vi "Configure Edge Trigger Source.vi"(0 "CS++Scope":refnum<class "CS++Scope.lvclass">, 5 "trigger source (CHANNEL1)":string(combo)="CHANNEL1" caption="trigger source (\"CHANNEL1\")", 7 "trigger slope (Positive)":i32(ring)=1 items=["Positive"=1, "Negative"=0], 9 "trigger level  (0.0 V)":dbl[unit] format="%.3f", 11 "error in (no error)":errorcluster) -> (4 "CS++Scope out":refnum<class "CS++Scope.lvclass">, 15 "error out":errorcluster)   [LabVIEW 2015, in "CS++Scope.lvlib" / "CS++Scope.lvclass"]
doc: "This VI configures the edge trigger. An edge trigger occurs when the trigger signal passes through the voltage threshold that you specify with the Trigger Level parameter and has the slope that you specify with the Trigger Slope parameter. \n\nNotes:\n (1) This VI affects instrument behavior only if the trigger type is\n IVISCOPE_VAL_EDGE_TRIGGER. Call the IviScope Configure Trigger and\n IviScope Configure Trigger Coupling VIs to set the trigger type and trigger coupling\n before calling this VI.\n (2) If the trigger source is one of the analog input channels, you must configure\n the vertical range, vertical offset, vertical coupling, probe attenuation, and the\n maximum input frequency before calling this VI."
uses:
  CS++Scope.lvclass
  CSPP_Core/Classes/CS++ProcessVariables/ProcessVariable/PV.lvclass
  PV-Enum.ctl
  CS++Scope.lvclass/CS++Scope.ctl
  CSPP_Core/Classes/CS++ProcessVariables/ProcessVariable/PV.lvclass/PV.ctl
  CSPP_Core/Classes/CS++ProcessVariables/ProcessVariable/Write Data.vi
  CSPP_Core/Classes/CS++ProcessVariables/ProcessVariable/Write Timestamp.vi
  CSPP_Core/Classes/CS++ProcessVariables/ProcessVariable/Write Quality.vi
  CSPP_Core/Classes/CS++ProcessVariables/ProcessVariable/Write status.vi
  CSPP_Core/Classes/CS++ProcessVariables/PVConnection/PVConnection.lvclass
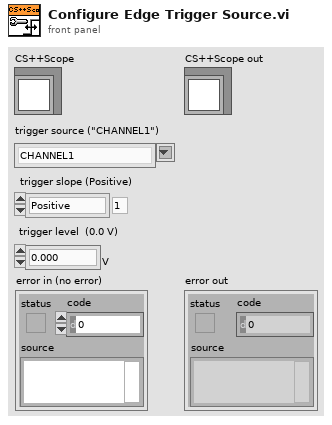
[diagram p1: front panel]
types:
  T1 = typedef "CS++Scope.lvlib/CS++Scope.lvclass/PV-Enum.ctl" = enum16{"ActualSampleRate", "TimePerRecord", "AcquisitionStartTime", "TriggerLevel", "GlitchWidth", "LowReference", "MidReference", "HighReference", "RuntLowThreshold", "RuntHighThreshold", "TriggerHoldoff", "WidthLowThreshold", "WidthHighThreshold", "AcquisitionStatus", "ActualRecordLength", "ActualSampleMode", "ACLineTriggerSlope", "MinRecordLength", "AcquisitionType", "TriggerSlope", "GlitchCondition", "GlitchPolarity", "InterpolationMethod", "NumberOfAverages", "NumberOfEnvelopes", "TriggerType", "TriggerCoupling", "TriggerModifier", "TVLineNumber", "TVEvent", "TVTriggerPolarity", "TVSignalFormat", "WidthCondition", "WidthPolarity", "MeasurementDone", "ContinousAcquisition", "TriggerSource", "Waveform", "ActualTimeIncrement"}
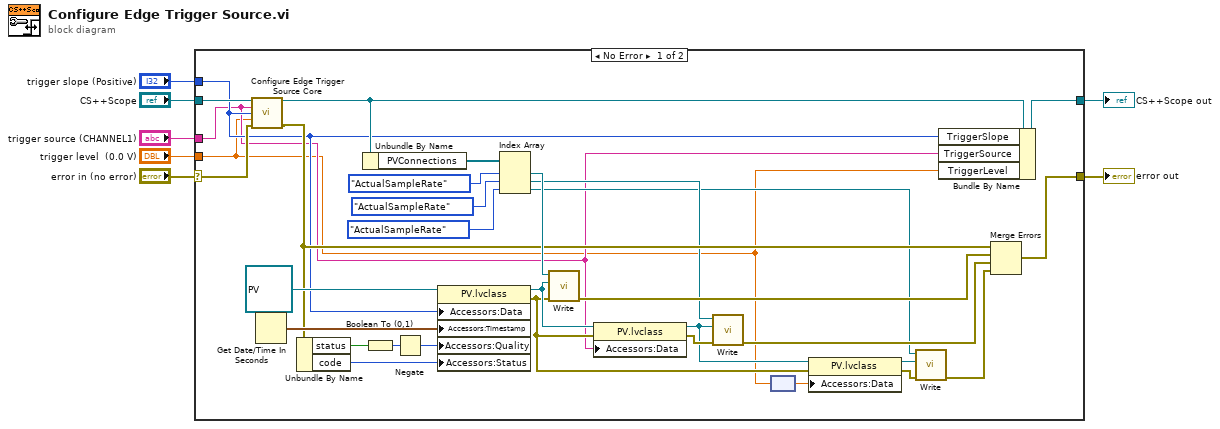
[diagram p0: block diagram]
diagram:
  n1 = case shown="No Error" "error in (no error)" {
    selector: "error in (no error)" -> [w13 w41]
    tunnel: [w12 w41] -> w6
    tunnel: [w14 w40] -> w2
    tunnel: "CS++Scope" -> [w15 w40]
    tunnel: "trigger source (CHANNEL1)" -> [w10 _]
    tunnel: "trigger level  (0.0 V)" -> [w9 _]
    tunnel: "trigger slope (Positive)" -> [w11 _]
    frame No Error {
      n2 = call-dynamic "Configure Edge Trigger Source Core.vi"("CS++Scope"=w15, "trigger source (CHANNEL1)"=w10, "trigger slope (Positive)"=w11, "trigger level  (0.0 V)"=w9, "error in (no error)"=w13) -> ("CS++Scope out"=w29:refnum<class "CS++Scope.lvclass">, "error out"=w28:errorcluster)  [unwired: 9 in]
      n3 = Get Date/Time In Seconds() -> (seconds since 1Jan1904=w34:timestamp)
      n4 = Unbundle By Name(w28) -> ("status"=w37:bool, "code"=w38:i32)
      n5 = Unbundle By Name(w29) -> ("PVConnections"=w33:refnum<class "PVConnection.lvclass">[])
      n6 = Boolean To (0,1)(Boolean=w37) -> (0, 1=w36:i16)
      n7 = Negate(x=w36) -> (-x=w35:i16)
      n8 = property class="PV.lvclass"(reference=refnum<class "PV.lvclass"> refnum ("CS++ProcessVariables.lvlib:PV.lvclass"), "Accessors:Data"=w11, "Accessors:Timestamp"=w34, "Accessors:Quality"=w35, "Accessors:Status"=w38) -> (reference out=w23:refnum<class "PV.lvclass">, error out=w19:errorcluster)  [unwired: 1 in]
      n9 = Index Array(array=w33, index #1=PV-Enum."ActualSampleRate" ("PV-Enum"), index #2=PV-Enum."ActualSampleRate" ("PV-Enum"), index #3=PV-Enum."ActualSampleRate" ("PV-Enum")) -> (element #1=w31:refnum<class "PVConnection.lvclass">, element #2=w21:refnum<class "PVConnection.lvclass">, element #3=w17:refnum<class "PVConnection.lvclass">)
      n10 = call "Write.vi"("error in (no error)"=w19, "PV"=w23, "PVConnection in"=w31) -> ("error out"=w30:errorcluster)  [unwired: 7 in, 1 out]
      n11 = property class="PV.lvclass"(reference=w23, error in=w19, "Accessors:Data"=w10) -> (reference out=w20:refnum<class "PV.lvclass">, error out=w22:errorcluster)
      n12 = call "Write.vi"("error in (no error)"=w22, "PV"=w20, "PVConnection in"=w21) -> ("error out"=w25:errorcluster)  [unwired: 7 in, 1 out]
      n13 = node(w9) -> (w8:dbl)
      n14 = property class="PV.lvclass"(reference=w20, error in=w19, "Accessors:Data"=w8) -> (reference out=w18:refnum<class "PV.lvclass">, error out=w16:errorcluster)
      n15 = call "Write.vi"("error in (no error)"=w16, "PV"=w18, "PVConnection in"=w17) -> ("error out"=w24:errorcluster)  [unwired: 7 in, 1 out]
      n16 = Bundle By Name(cluster=w29, "TriggerSlope"=w11, "TriggerSource"=w10, "TriggerLevel"=w9) -> (w14:refnum<class "CS++Scope.lvclass">)
      n17 = Merge Errors(w28, w30, w25, w24) -> (w12:errorcluster)
    }
    frame Error {
    }
  }
  "error out" <- w6
  "CS++Scope out" <- w2
